vi "create.TradeLong.vi"(8 "error in":errorcluster, 10 "TradeLong.Parameters":T1={"Time Offset"=447000, "Order Id"="ORID0001", "Execution Id"="EXE_ID_1", "Quantity"=20000, "Price"=0.905, "Side Indicator"="B", "Symbol"="AAPL"}, 11 "TradeLong in":refnum<class "TradeLong.lvclass">) -> (0 "error out":errorcluster, 3 "TradeLong out":refnum<class "TradeLong.lvclass">)   [LabVIEW 2020, in "TradeLong.lvclass"]
uses:
  TradeLong.lvclass
  TradeLong.Parameters.ctl
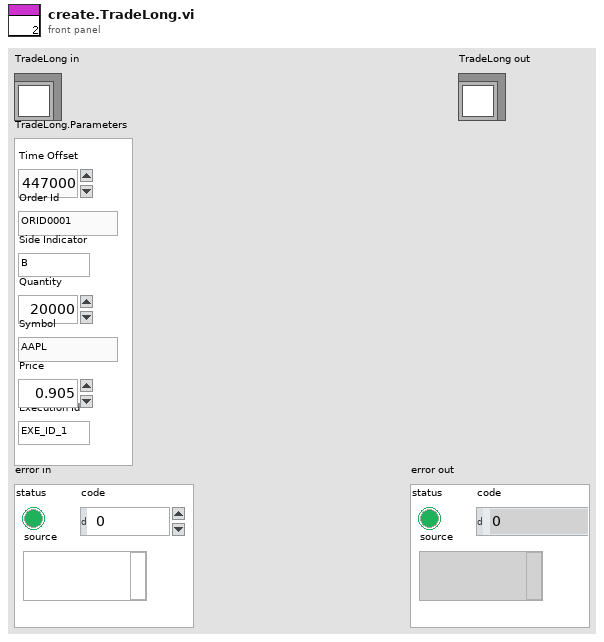
[diagram p1: front panel]
types:
  T1 = typedef "TradeLong.lvclass/TradeLong.Parameters.ctl" = cluster{"Time Offset":u32, "Order Id":string, "Execution Id":string, "Quantity":u32, "Price":dbl, "Side Indicator":string, "Symbol":string}
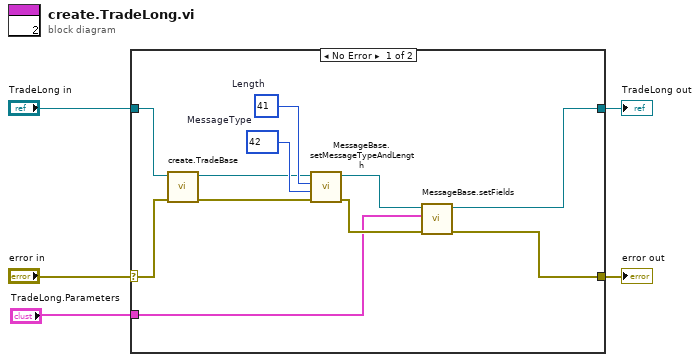
[diagram p0: block diagram]
diagram:
  n1 = case shown="No Error" "error in" {
    selector: "error in" -> [w11 w18]
    tunnel: [w7 w18] -> w4
    tunnel: [w6 w17] -> w2
    tunnel: "TradeLong in" -> [w12 w17]
    tunnel: "TradeLong.Parameters" -> [w8 _]
    frame No Error {
      w15 = u8 42  # MessageType
      w16 = u8 41  # Length
      n2 = call-dynamic "create.TradeBase.vi"("error in (no error)"=w11, "TradeBase in"=w12) -> ("error out"=w14:errorcluster, "TradeBase out"=w13:refnum<class "TradeLong.lvclass">)  [unwired: 8 in]
      n3 = call-dynamic "MessageBase.setMessageTypeAndLength.vi"("error in (no error)"=w14, "MessageType"=w15, "Length"=w16, "MessageBase in"=w13) -> ("error out"=w9:errorcluster, "MessageBase out"=w10:refnum<class "TradeLong.lvclass">)  [unwired: 6 in]
      n4 = call-dynamic "MessageBase.setFields.vi"("error in (no error)"=w9, "Cluster (dup)"=w8, "MessageBase in"=w10) -> ("error out"=w7:errorcluster, "MessageBase out"=w6:refnum<class "TradeLong.lvclass">)  [unwired: 7 in]
    }
    frame Error {
    }
  }
  "error out" <- w4
  "TradeLong out" <- w2
